vi "Main.vi"() -> ()   [LabVIEW 2020, in "Application.lvlib"]
doc: "This VI is the main application VI in the Delacor QMH project template. This application VI is implemented as a simple state machine, which communicates with two different Delacor QMH modules.\n_____\nBased on DQMH Project Template 6.1.0.93."
uses:
  Application.lvlib
  Application Data--cluster.ctl
  State--enum.ctl
  <vilib>/Utility/error.llb/DialogType.ctl
  Cloneable Module/Cloneable Module.lvlib
  Singleton Module/Singleton Module.lvlib
panel:
  in  "About DQMH":bool
  out "version":string
  in  "Hide Singleton Module Module":bool
  in  "Show Singleton Module Module":bool
  in  "Hide Cloneable Module Module":bool
  in  "Show Cloneable Module Module":bool
  in  "Stop Cloneable Module Module":bool
  in  "Stop Singleton Module Module":bool
  in  "Start Singleton Module Module":bool
  out "Active Cloneable Module Modules":string[](array[string])
  in  "Start New Instance Cloneable Module Module":bool
  in  "Select Cloneable Module Module Instance":i32(ring)=-1 items=["All"=-1, "1"=1]
  in  "Singleton Module Module: Do Something Else":dbl caption="Do Something Else"
  in  "Singleton Module Module: Do Something":bool
  out "Singleton Module Running?":bool
  out "Status":string
  in  "Cloneable Module Module: Do Something Else":dbl caption="Do Something Else to Selected Module"
  in  "Cloneable Module Module: Do Something":bool caption="Do Something to Selected Module"
  # "This top-level application allows you to launch and control a singleton module, and multiple instances of a cloneable module."
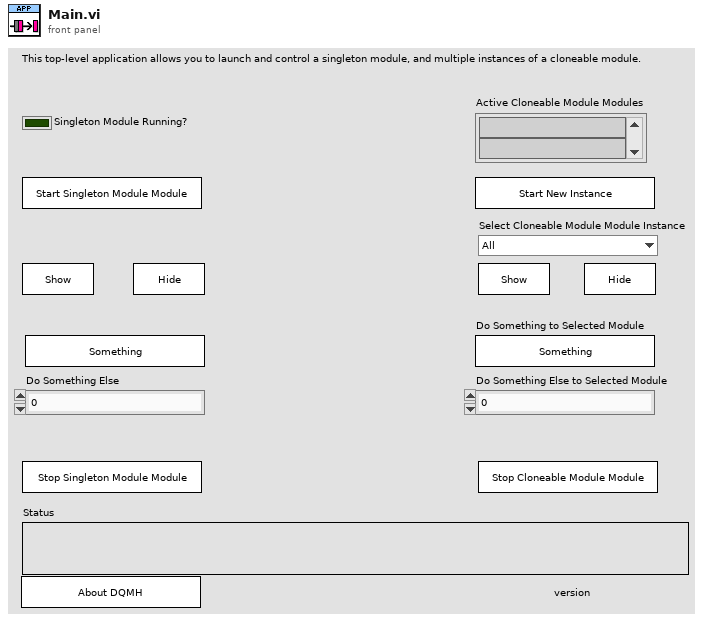
[diagram p1: front panel]
types:
  T1 = typedef "Application.lvlib/State--enum.ctl" = enum16{"Initialize", "Initialize Panel", "UI Interlocks", "Update Status", "Wait for Event", "Exit"}
  T2 = typedef "Application.lvlib/Application Data--cluster.ctl" = cluster{"Status":string, "Singleton Controls":refnum<vi>[], "Cloneable Controls":refnum<vi>[], "Module Ring Value":i32}
  T3 = typedef "Cloneable Module.lvlib/Broadcast Events--cluster.ctl" = cluster{"Module Did Init":refnum<user-event>, "Status Updated":refnum<user-event>, "Error Reported":refnum<user-event>, "Did Something":refnum<user-event>, "Module Did Stop":refnum<user-event>, "Update Module Execution Status":refnum<user-event>}
  T4 = typedef "Singleton Module.lvlib/Broadcast Events--cluster.ctl" = cluster{"Module Did Init":refnum<user-event>, "Status Updated":refnum<user-event>, "Error Reported":refnum<user-event>, "Did Something":refnum<user-event>, "Module Did Stop":refnum<user-event>, "Update Module Execution Status":refnum<user-event>}
  T5 = enum8{"Enabled", "Disabled", "Disabled and Grayed Out"}
  T6 = typedef "DialogType.ctl" = u16
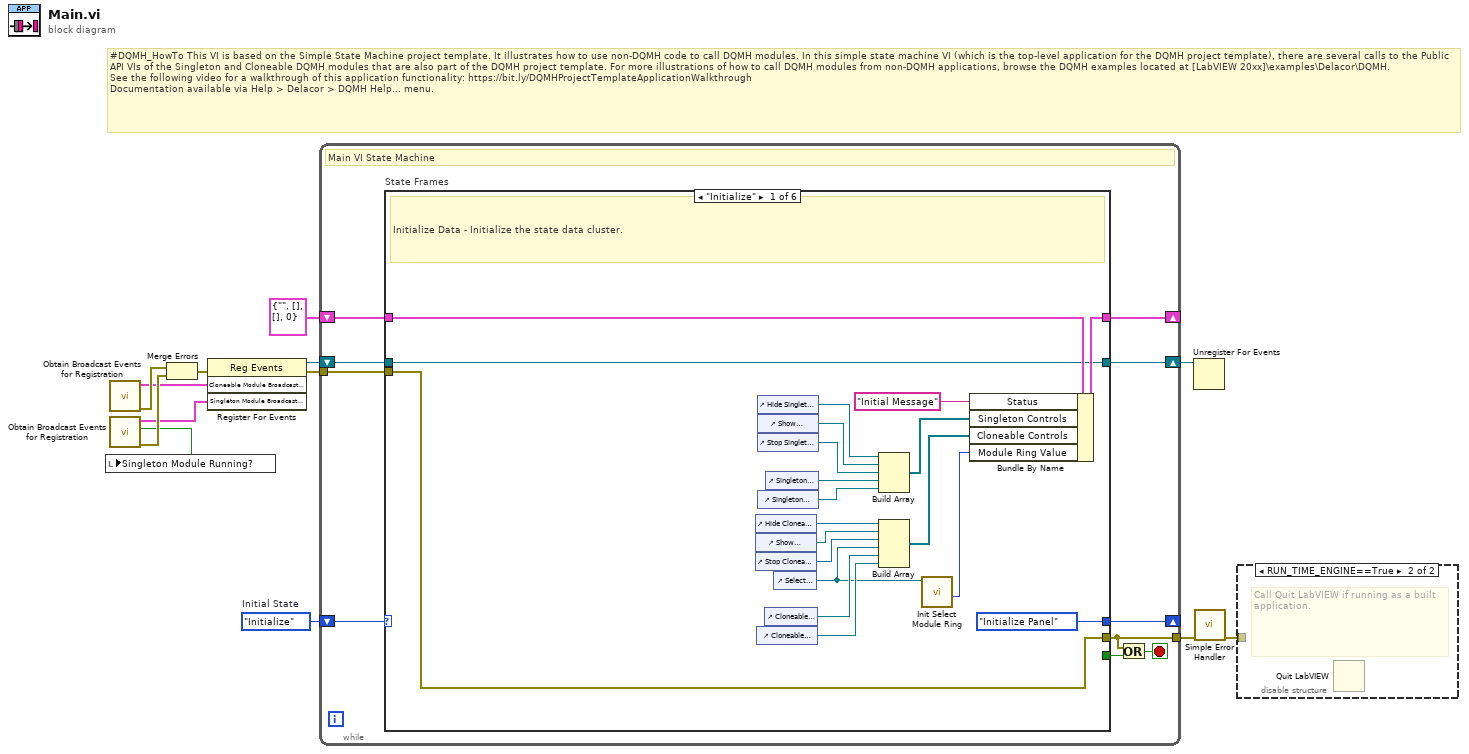
[diagram p0: block diagram]
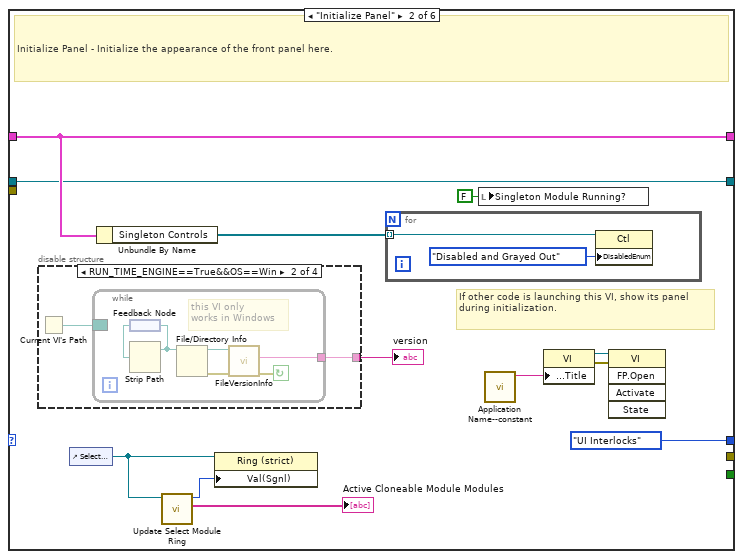
[diagram p2: hidden frame]
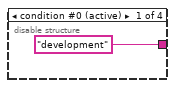
[diagram p3: hidden frame]
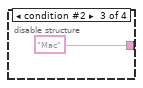
[diagram p4: hidden frame]
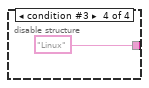
[diagram p5: hidden frame]
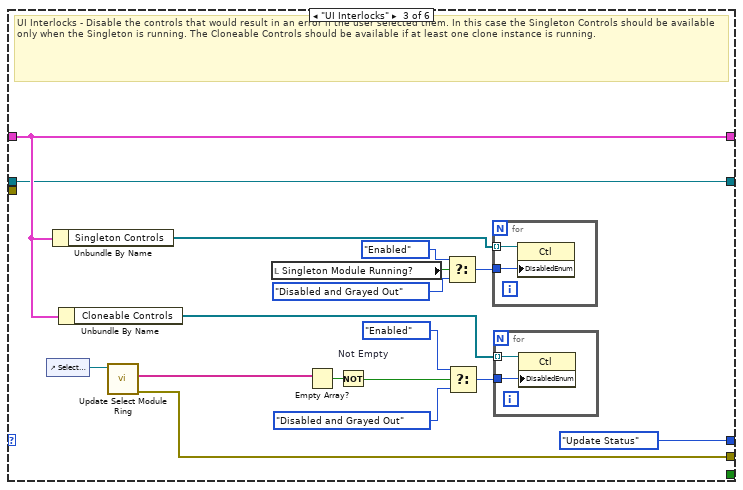
[diagram p6: hidden frame]
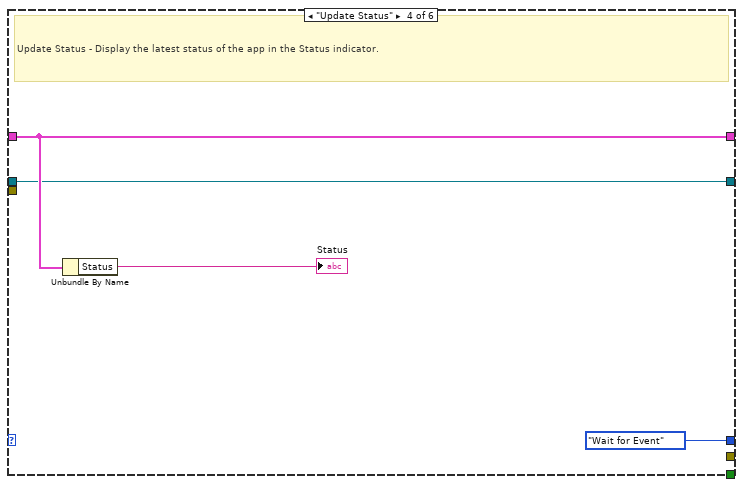
[diagram p7: hidden frame]
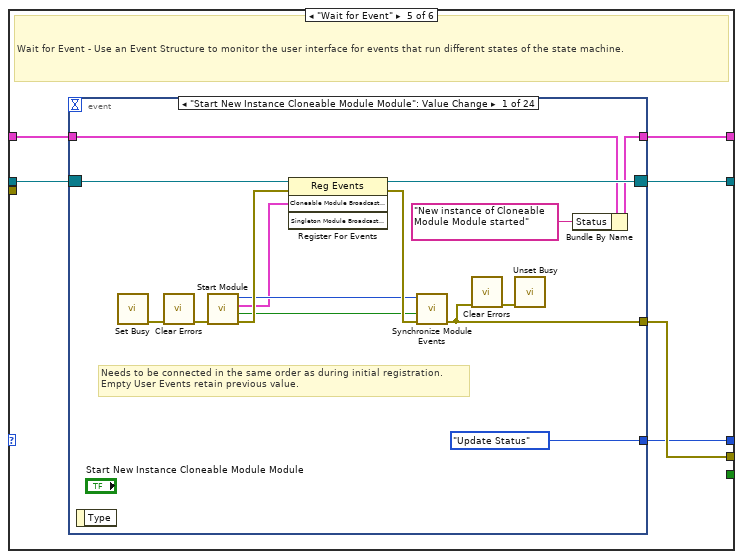
[diagram p8: hidden frame]
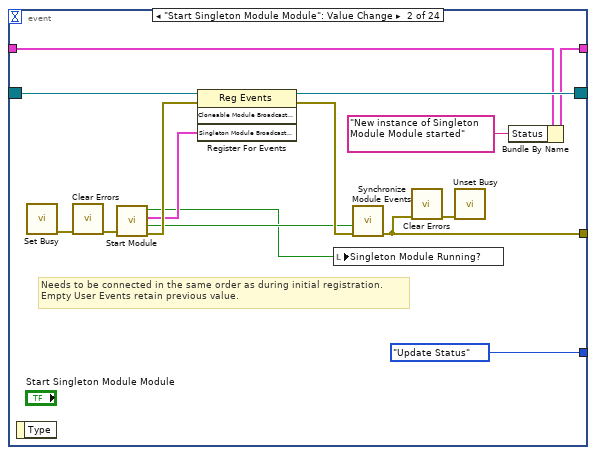
[diagram p9: hidden frame]
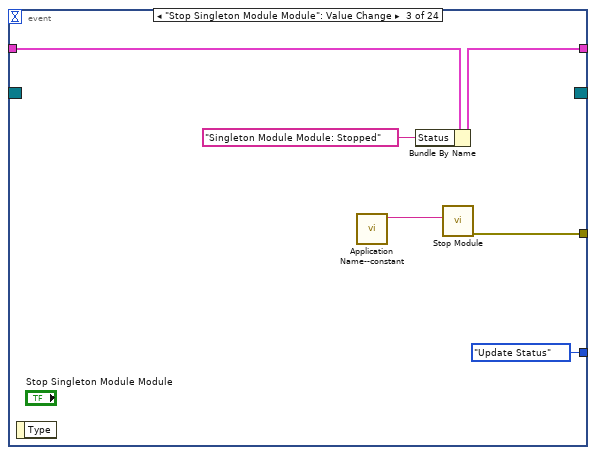
[diagram p10: hidden frame]
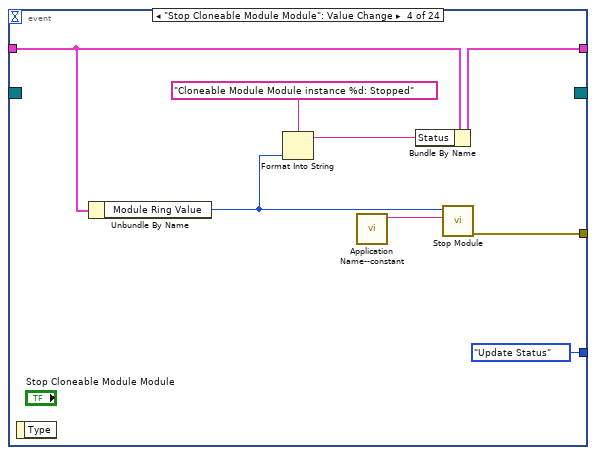
[diagram p11: hidden frame]
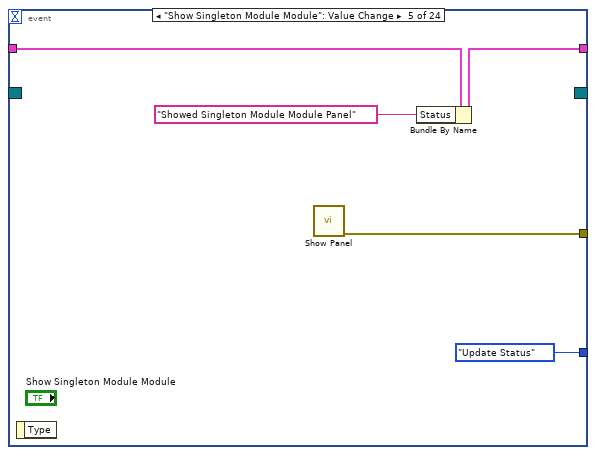
[diagram p12: hidden frame]
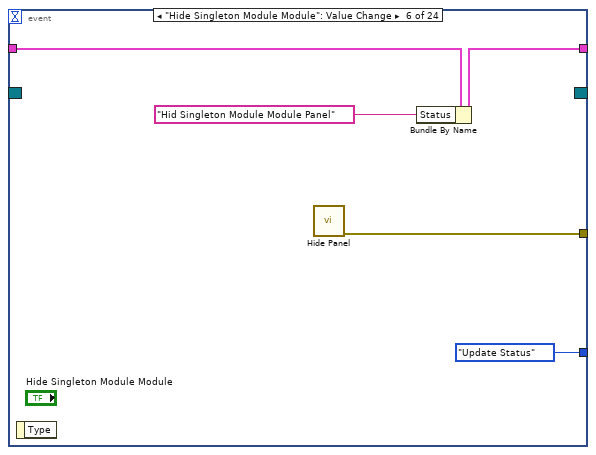
[diagram p13: hidden frame]
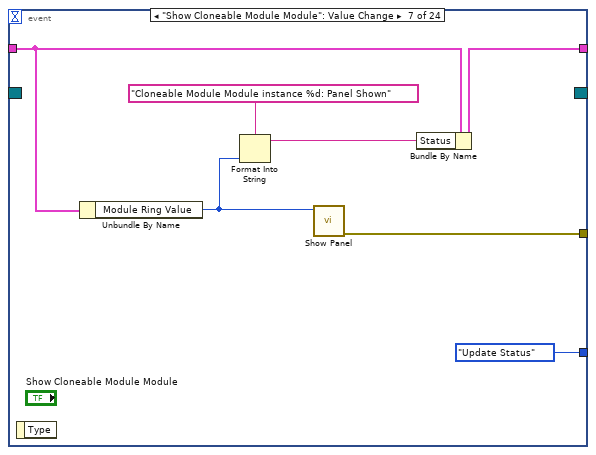
[diagram p14: hidden frame]
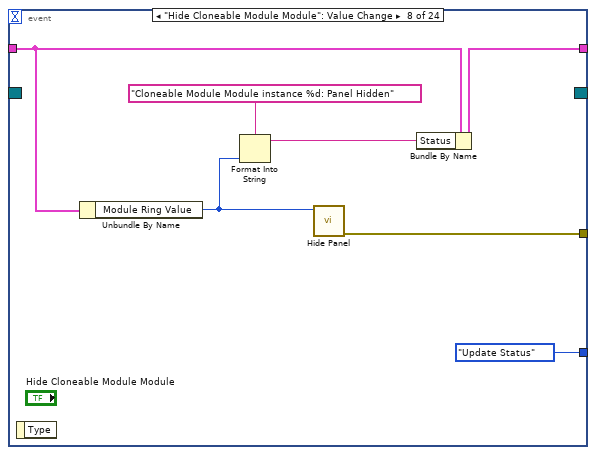
[diagram p15: hidden frame]
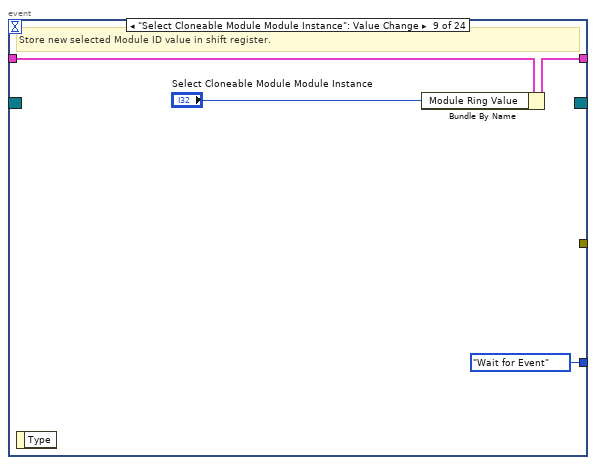
[diagram p16: hidden frame]
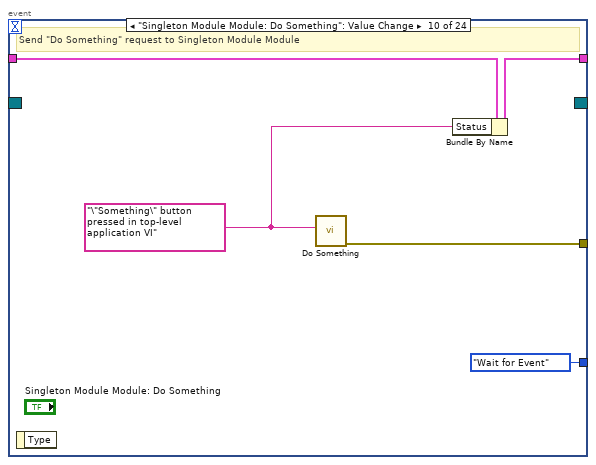
[diagram p17: hidden frame]
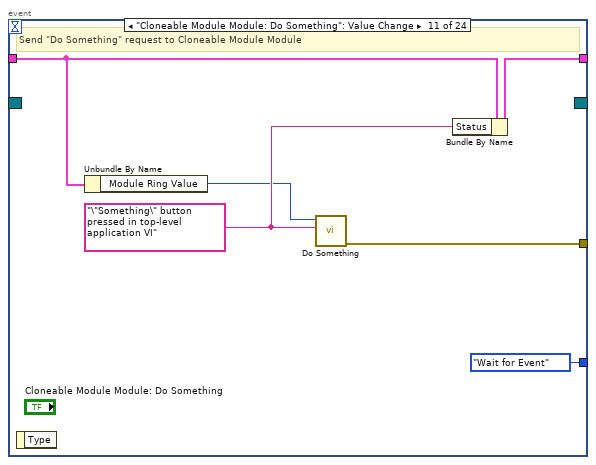
[diagram p18: hidden frame]
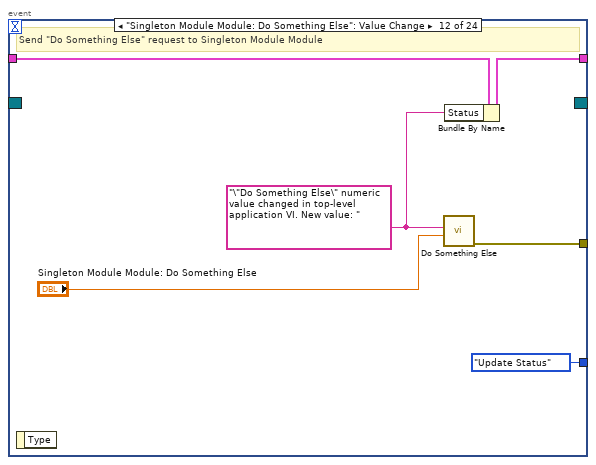
[diagram p19: hidden frame]
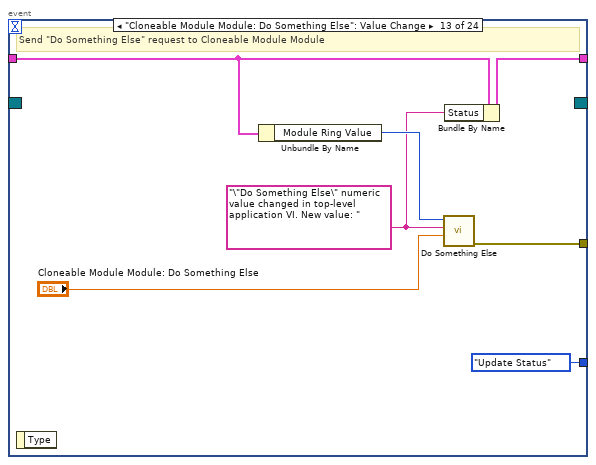
[diagram p20: hidden frame]
diagram:
  w4 = State--enum."Initialize"  # Initial State
  # "#DQMH_HowTo This VI is based on the Simple State Machine project template. It illustrates how to use non-DQMH code to call DQMH modules. In this simple state machine VI (which is the top-level application for the DQMH project template), there are several calls to the Public API VIs of the Singleton and Cloneable DQMH modules that are also part of the DQMH project template. For more illustrations of how to call DQMH modules from non-DQMH applications, browse the DQMH examples located at [LabVIEW 20xx]\\examples\\Delacor\\DQMH.\nSee the following video for a walkthrough of this application functionality: https://bit.ly/DQMHProjectTemplateApplicationWalkthrough\nDocumentation available via Help > Delacor > DQMH Help... menu."
  n1 = call "Obtain Broadcast Events for Registration.vi"() -> ("error out"=w9:errorcluster, "Cloneable Module Broadcast Events"=w6:T3)  [unwired: 9 in, 1 out]
  n2 = call "Obtain Broadcast Events for Registration.vi"() -> ("error out"=w8:errorcluster, "Already running?"=w1:bool, "Singleton Module Broadcast Events"=w5:T4)  [unwired: 9 in]
  n3 = local write "Singleton Module Running?"(w1) -> ()
  n4 = Merge Errors(w9, w8) -> (w10:errorcluster)
  n5 = register-events(error in=w10, w6, w5) -> (reference out=w3:refnum<event-registration>, error out=w11:errorcluster)  [unwired: 1 in]
  n6 = while {
    shift-right: [w20] -> _
    shift-left: T2 {"Status"="", "Singleton Controls"=[], "Cloneable Controls"=[], "Module Ring Value"=0} ("Data Cluster") -> [w21]
    tunnel: [w23] -> w13
    shift-right: [w16] -> _
    shift-left: w4 -> [w18]
    shift-right: [w14] -> w2
    shift-left: w3 -> [w15]
    tunnel: w11 -> [w22]
    stop <- w17 stop-if-true
    # "Main VI State Machine"
    n7 = case "State Frames" shown="\"Initialize\"" w18 {
      tunnel: [w43 _ w85 _ w99 w277] -> w23
      tunnel: w21 -> [w42 w52 w73 w93 w96 w274]
      tunnel: [w41 w52 w73 w93 w95 w274] -> w20
      tunnel: [_ _ _ _ _ w273] -> w19
      tunnel: [State--enum."Initialize Panel" ("State") State--enum."UI Interlocks" ("State") State--enum."Update Status" ("State") State--enum."Wait for Event" ("State") w94 State--enum."Exit" ("State")] -> w16
      tunnel: w15 -> [w24 w49 w69 w90 w98 w271]
      tunnel: [w24 w49 w69 w90 w97 w271] -> w14
      tunnel: w22 -> [w43 _ _ _ _ _]
      frame "Initialize" {
        # "Initialize Data - Initialize the state data cluster."
        n8 = control-ref of="Hide Cloneable Module Module"() -> (w33:refnum<vi>)
        n9 = control-ref of="Show Cloneable Module Module"() -> (w32:refnum<vi>)
        n10 = control-ref of="Stop Cloneable Module Module"() -> (w31:refnum<vi>)
        n11 = control-ref of="Cloneable Module Module: Do Something"() -> (w28:refnum<vi>)
        n12 = control-ref of="Hide Singleton Module Module"() -> (w39:refnum<vi>)
        n13 = control-ref of="Show Singleton Module Module"() -> (w38:refnum<vi>)
        n14 = control-ref of="Stop Singleton Module Module"() -> (w37:refnum<vi>)
        n15 = control-ref of="Singleton Module Module: Do Something"() -> (w35:refnum<vi>)
        n16 = control-ref of="Cloneable Module Module: Do Something Else"() -> (w29:refnum<vi>)
        n17 = control-ref of="Singleton Module Module: Do Something Else"() -> (w36:refnum<vi>)
        n18 = control-ref of="Select Cloneable Module Module Instance"() -> (w26:refnum<vi>)
        n19 = Build Array(w39, w38, w37, w36, w35) -> (w34:refnum<vi>[])
        n20 = Build Array(w33, w32, w31, w26, w29, w28) -> (w30:refnum<vi>[])
        n21 = call "Init Select Module Ring.vi"("Select Module Ring Ref"=w26) -> ("Module Ring Value"=w25:i32)  [unwired: 8 in, 2 out]
        n22 = Bundle By Name(cluster=w42, "Status"="Initial Message" ("Initial Message"), "Singleton Controls"=w34, "Cloneable Controls"=w30, "Module Ring Value"=w25) -> (w41:T2)
      }
      frame "Initialize Panel" {
        # "If other code is launching this VI, show its panel during initialization."
        # "Initialize Panel - Initialize the appearance of the front panel here."
        n23 = disable-structure "Conditional Disable Structure" shown="RUN_TIME_ENGINE==True&&OS==Win" {
          disable-tunnel: ["development" w57 "Mac" "Linux"] -> w46
          frame condition #0 (active) {
          }
          frame condition #1 {
            n24 = Current VI's Path() -> (path=w58:path)
            n25 = while {
              border: w58 -> [_]
              tunnel: [w59] -> w57
              stop <- w63 continue-if-true
              # "this VI only \nworks in Windows"
              n26 = feedback #1() -> (w62:path)
              n27 = Strip Path(path=w62) -> (stripped path=w61:path)  [unwired: 1 out]
              n28 = feedback-in #1(w61) -> ()
              n29 = File/Directory Info(path=w61) -> (path out=w60:path, error out=w64:errorcluster)  [unwired: 1 in, 5 out]
              n30 = call <vilib>:"FileVersionInfo.vi"("error in (no error)"=w64, "Application Path in"=w60) -> ("error out"=w63:errorcluster, "File Version Info"=w59:string)  [unwired: 6 in, 2 out]
            }
          }
          frame condition #2 {
          }
          frame condition #3 {
          }
        }
        "version" <- w46
        n31 = control-ref of="Select Cloneable Module Module Instance"() -> (w48:refnum<vi>)
        n32 = Unbundle By Name(w52) -> ("Singleton Controls"=w51:refnum<vi>[])
        n33 = call "Update Select Module Ring.vi"("Select Module Ring Ref"=w48) -> ("Active Modules (Array)"=→"Active Cloneable Module Modules":string[], "New Module Ring Value"=w47:i32)  [unwired: 8 in, 1 out]
        n34 = property on="Property Node" class="Ring (strict)"(reference=w48, "Val(Sgnl)"=w47) -> ()  [unwired: 1 in, 2 out]
        n35 = for {
          tunnel: w51 -> [w68] mode=indexing
          n36 = property on="Property Node" class="Ctl"(reference=w68, "DisabledEnum"=T5."Disabled and Grayed Out" ("Disabled")) -> ()  [unwired: 1 in, 2 out]
        }
        n37 = local write "Singleton Module Running?"(FALSE ("My Singleton Module Init?")) -> ()
        n38 = call "Application Name--constant.vi"() -> ("Application Name"=w45:string)  [unwired: 11 in]
        n39 = property on="Property Node" class="VI"("Front Panel.Title"=w45) -> (reference out=w44:refnum<vi>, error out=w55:errorcluster)  [unwired: 2 in]
        n40 = invoke class="VI" method="FP.Open"(reference=w44, error in=w55) -> ()  [unwired: 3 in, 5 out]
      }
      frame "UI Interlocks" {
        # "UI Interlocks - Disable the controls that would result in an error if the user selected them. In this case the Singleton Controls should be available only when the Singleton is running. The Cloneable Controls should be available if at least one clone instance is running."
        n41 = control-ref of="Select Cloneable Module Module Instance"() -> (w84:refnum<vi>)
        n42 = Unbundle By Name(w73) -> ("Singleton Controls"=w78:refnum<vi>[])
        n43 = Unbundle By Name(w73) -> ("Cloneable Controls"=w72:refnum<vi>[])
        n44 = call "Update Select Module Ring.vi"("Select Module Ring Ref"=w84) -> ("error out"=w85:errorcluster, "Active Modules (Array)"=w83:string[])  [unwired: 8 in, 1 out]
        n45 = local read "Singleton Module Running?"() -> (w77:bool)
        n46 = Empty Array?(array=w83) -> (empty?=w82:bool)
        n47 = Not "Not Empty"(x=w82) -> (.not. x?=w71:bool)
        n48 = Select(t=T5."Enabled" ("Disabled"), s=w77, f=T5."Disabled and Grayed Out" ("Disabled")) -> (s? t:f=w79:T5)
        n49 = Select(t=T5."Enabled" ("Disabled"), s=w71, f=T5."Disabled and Grayed Out" ("Disabled")) -> (s? t:f=w76:T5)
        n50 = for {
          tunnel: w78 -> [w89] mode=indexing
          tunnel: w79 -> [w88]
          n51 = property on="Property Node" class="Ctl"(reference=w89, "DisabledEnum"=w88) -> ()  [unwired: 1 in, 2 out]
        }
        n52 = for {
          tunnel: w72 -> [w87] mode=indexing
          tunnel: w76 -> [w86]
          n53 = property on="Property Node" class="Ctl"(reference=w87, "DisabledEnum"=w86) -> ()  [unwired: 1 in, 2 out]
        }
      }
      frame "Update Status" {
        # "Update Status - Display the latest status of the app in the Status indicator."
        n54 = Unbundle By Name(w93) -> ("Status"=→"Status":string)
      }
      frame "Wait for Event" {
        # "Wait for Event - Use an Event Structure to monitor the user interface for events that run different states of the state machine."
        n55 = event shown="[0] \"Start New Instance Cloneable Module Module\": Value Change" {
          selector: w98 -> [w106 w122 _ _ _ _ _ _ _ _ _ _ _ _ _ _ _ _ _ _ _ _ _ _]
          dyn-events: [w105 w121 _ _ _ _ _ _ _ _ _ _ _ _ _ _ _ _ _ _ _ _ _ _] -> w97
          timeout: _ -> [_ _ _ _ _ _ _ _ _ _ _ _ _ _ _ _ _ _ _ _ _ _ _ _]
          tunnel: [w114 w129 w135 w143 w148 w153 w160 w167 _ w176 w182 w188 w195 w203 w208 w212 _ _ _ _ w254 _ _ w265] -> w99
          tunnel: [w101 w118 w131 w140 w146 w151 w159 w166 w169 w174 w181 w186 w194 w197 w205 w211 w214 w219 w234 w243 w247 w258 w263 w267] -> w95
          tunnel: w96 -> [w102 w119 w132 w139 w147 w152 w157 w164 w170 w175 w178 w187 w192 w197 w205 w211 w215 w220 w235 w244 w250 w259 w263 w267]
          tunnel: [State--enum."Update Status" ("State") State--enum."Update Status" ("State") State--enum."Update Status" ("State") State--enum."Update Status" ("State") State--enum."Update Status" ("State") State--enum."Update Status" ("State") State--enum."Update Status" ("State") State--enum."Update Status" ("State") State--enum."Wait for Event" ("State") State--enum."Wait for Event" ("State") State--enum."Wait for Event" ("State") State--enum."Update Status" ("State") State--enum."Update Status" ("State") State--enum."UI Interlocks" ("State") State--enum."UI Interlocks" ("State") State--enum."UI Interlocks" ("State") State--enum."Update Status" ("State") State--enum."Update Status" ("State") State--enum."Update Status" ("State") State--enum."Update Status" ("State") State--enum."UI Interlocks" ("State") State--enum."UI Interlocks" ("State") State--enum."Exit" ("State") State--enum."Wait for Event" ("State")] -> w94
          event "Start New Instance Cloneable Module Module": Value Change {
            # "Needs to be connected in the same order as during initial registration.\nEmpty User Events retain previous value."
            n56 = event-data() -> ()  [unwired: 1 in, 1 out]
            n57 = call <vilib>:"Set Busy.vi"() -> ("error out"=w110:errorcluster)  [unwired: 10 in, 1 out]
            n58 = call <vilib>:"Clear Errors.vi"("error in (no error)"=w110) -> ("error out"=w111:errorcluster)  [unwired: 5 in, 1 out]
            n59 = call "Start Module.vi"("error in"=w111) -> ("error out"=w113:errorcluster, "Wait for Event Sync?"=w108:bool, "Cloneable Module Broadcast Events"=w104:T3, "Module ID"=w107:i32)  [unwired: 7 in]
            n60 = register-events(reference=w106, error in=w113, w104) -> (reference out=w105:refnum<event-registration>, error out=w112:errorcluster)  [unwired: 1 in]
            n61 = call "Synchronize Module Events.vi"("error in"=w112, "Wait for Event Sync?"=w108, "Module ID in"=w107) -> ("error out"=w114:errorcluster)  [unwired: 7 in, 1 out]
            n62 = call <vilib>:"Clear Errors.vi"("error in (no error)"=w114) -> ("error out"=w109:errorcluster)  [unwired: 5 in, 1 out]
            n63 = call <vilib>:"Unset Busy.vi"("error in (no error)"=w109) -> ()  [unwired: 10 in, 1 out]
            n64 = Bundle By Name(cluster=w102, "Status"="New instance of Cloneable Module Module started") -> (w101:T2)
          }
          event "Start Singleton Module Module": Value Change {
            # "Needs to be connected in the same order as during initial registration.\nEmpty User Events retain previous value."
            n65 = event-data() -> ()  [unwired: 1 in, 1 out]
            n66 = call <vilib>:"Set Busy.vi"() -> ("error out"=w125:errorcluster)  [unwired: 10 in, 1 out]
            n67 = call <vilib>:"Clear Errors.vi"("error in (no error)"=w125) -> ("error out"=w126:errorcluster)  [unwired: 5 in, 1 out]
            n68 = call "Start Module.vi"("error in"=w126) -> ("error out"=w128:errorcluster, "Wait for Event Sync?"=w123:bool, "Singleton Module Broadcast Events"=w116:T4, "Module Was Already Running?"=w115:bool)  [unwired: 7 in]
            n69 = register-events(reference=w122, error in=w128, w116) -> (reference out=w121:refnum<event-registration>, error out=w127:errorcluster)  [unwired: 1 in]
            n70 = local write "Singleton Module Running?"(w115) -> ()
            n71 = call "Synchronize Module Events.vi"("error in"=w127, "Wait for Event Sync?"=w123) -> ("error out"=w129:errorcluster)  [unwired: 9 in]
            n72 = call <vilib>:"Clear Errors.vi"("error in (no error)"=w129) -> ("error out"=w124:errorcluster)  [unwired: 5 in, 1 out]
            n73 = call <vilib>:"Unset Busy.vi"("error in (no error)"=w124) -> ()  [unwired: 10 in, 1 out]
            n74 = Bundle By Name(cluster=w119, "Status"="New instance of Singleton Module Module started") -> (w118:T2)
          }
          event "Stop Singleton Module Module": Value Change {
            n75 = event-data() -> ()  [unwired: 1 in, 1 out]
            n76 = call "Application Name--constant.vi"() -> ("Application Name"=w133:string)  [unwired: 11 in]
            n77 = Bundle By Name(cluster=w132, "Status"="Singleton Module Module: Stopped" ("Message")) -> (w131:T2)
            n78 = call "Stop Module.vi"("Origin"=w133) -> ("error out"=w135:errorcluster)  [unwired: 10 in]
          }
          event "Stop Cloneable Module Module": Value Change {
            n79 = event-data() -> ()  [unwired: 1 in, 1 out]
            n80 = Unbundle By Name(w139) -> ("Module Ring Value"=w136:i32)
            n81 = Format Into String(format string="Cloneable Module Module instance %d: Stopped" ("Message"), w136) -> (resulting string=w137:string)  [unwired: 2 in, 1 out]
            n82 = call "Application Name--constant.vi"() -> ("Application Name"=w141:string)  [unwired: 11 in]
            n83 = Bundle By Name(cluster=w139, "Status"=w137) -> (w140:T2)
            n84 = call "Stop Module.vi"("Origin"=w141, "Module ID"=w136) -> ("error out"=w143:errorcluster)  [unwired: 9 in]
          }
          event "Show Singleton Module Module": Value Change {
            n85 = event-data() -> ()  [unwired: 1 in, 1 out]
            n86 = call "Show Panel.vi"() -> ("error out"=w148:errorcluster)  [unwired: 11 in]
            n87 = Bundle By Name(cluster=w147, "Status"="Showed Singleton Module Module Panel" ("Message")) -> (w146:T2)
          }
          event "Hide Singleton Module Module": Value Change {
            n88 = event-data() -> ()  [unwired: 1 in, 1 out]
            n89 = call "Hide Panel.vi"() -> ("error out"=w153:errorcluster)  [unwired: 11 in]
            n90 = Bundle By Name(cluster=w152, "Status"="Hid Singleton Module Module Panel" ("Message")) -> (w151:T2)
          }
          event "Show Cloneable Module Module": Value Change {
            n91 = event-data() -> ()  [unwired: 1 in, 1 out]
            n92 = Unbundle By Name(w157) -> ("Module Ring Value"=w155:i32)
            n93 = Format Into String(format string="Cloneable Module Module instance %d: Panel Shown" ("Message"), w155) -> (resulting string=w154:string)  [unwired: 2 in, 1 out]
            n94 = call "Show Panel.vi"("Module ID"=w155) -> ("error out"=w160:errorcluster)  [unwired: 10 in]
            n95 = Bundle By Name(cluster=w157, "Status"=w154) -> (w159:T2)
          }
          event "Hide Cloneable Module Module": Value Change {
            n96 = event-data() -> ()  [unwired: 1 in, 1 out]
            n97 = Unbundle By Name(w164) -> ("Module Ring Value"=w162:i32)
            n98 = Format Into String(format string="Cloneable Module Module instance %d: Panel Hidden" ("Message"), w162) -> (resulting string=w161:string)  [unwired: 2 in, 1 out]
            n99 = call "Hide Panel.vi"("Module ID"=w162) -> ("error out"=w167:errorcluster)  [unwired: 10 in]
            n100 = Bundle By Name(cluster=w164, "Status"=w161) -> (w166:T2)
          }
          event "Select Cloneable Module Module Instance": Value Change {
            # "Store new selected Module ID value in shift register."
            n101 = event-data() -> ()  [unwired: 1 in, 1 out]
            n102 = Bundle By Name(cluster=w170, "Module Ring Value"="Select Cloneable Module Module Instance") -> (w169:T2)
          }
          event "Singleton Module Module: Do Something": Value Change {
            w173 = "\"Something\" button pressed in top-level application VI" ("\"Do Something Else\" button pressed")
            # "Send \"Do Something\" request to Singleton Module Module"
            n103 = event-data() -> ()  [unwired: 1 in, 1 out]
            n104 = call "Do Something.vi"("Do Something Message"=w173) -> ("error out"=w176:errorcluster)  [unwired: 10 in]
            n105 = Bundle By Name(cluster=w175, "Status"=w173) -> (w174:T2)
          }
          event "Cloneable Module Module: Do Something": Value Change {
            w180 = "\"Something\" button pressed in top-level application VI" ("\"Do Something Else\" button pressed")
            # "Send \"Do Something\" request to Cloneable Module Module"
            n106 = event-data() -> ()  [unwired: 1 in, 1 out]
            n107 = Unbundle By Name(w178) -> ("Module Ring Value"=w177:i32)
            n108 = call "Do Something.vi"("Do Something Message"=w180, "Module ID"=w177) -> ("error out"=w182:errorcluster)  [unwired: 9 in]
            n109 = Bundle By Name(cluster=w178, "Status"=w180) -> (w181:T2)
          }
          event "Singleton Module Module: Do Something Else": Value Change {
            w183 = "\"Do Something Else\" numeric value changed in top-level application VI. New value: " ("\"Do Something Else\" button pressed")
            # "Send \"Do Something Else\" request to Singleton Module Module"
            n110 = event-data() -> ()  [unwired: 1 in, 1 out]
            n111 = call "Do Something Else.vi"("X"="Singleton Module Module: Do Something Else", "Do Something Else Message"=w183) -> ("error out"=w188:errorcluster)  [unwired: 9 in]
            n112 = Bundle By Name(cluster=w187, "Status"=w183) -> (w186:T2)
          }
          event "Cloneable Module Module: Do Something Else": Value Change {
            w189 = "\"Do Something Else\" numeric value changed in top-level application VI. New value: " ("\"Do Something Else\" button pressed")
            # "Send \"Do Something Else\" request to Cloneable Module Module"
            n113 = event-data() -> ()  [unwired: 1 in, 1 out]
            n114 = Unbundle By Name(w192) -> ("Module Ring Value"=w191:i32)
            n115 = call "Do Something Else.vi"("X"="Cloneable Module Module: Do Something Else", "Do Something else Message"=w189, "Module ID"=w191) -> ("error out"=w195:errorcluster)  [unwired: 8 in]
            n116 = Bundle By Name(cluster=w192, "Status"=w189) -> (w194:T2)
          }
          event User Event {
            # "A new instance of Cloneable Module Module has broadcast that is has been initialized"
            n117 = event-data() -> ("Info"=w201:string, "Module ID"=w196:i32)  [unwired: 1 in]
            n118 = local write "Status"(w201) -> ()
            n119 = control-ref of="Select Cloneable Module Module Instance"() -> (w200:refnum<vi>)
            n120 = call "Update Select Module Ring.vi"("Select Module Ring Ref"=w200) -> ("error out"=w202:errorcluster, "Active Modules (Array)"=w199:string[])  [unwired: 8 in, 1 out]
            n121 = local write "Active Cloneable Module Modules"(w199) -> ()
            n122 = call "Show Panel.vi"("error in (no error)"=w202, "Module ID"=w196) -> ("error out"=w203:errorcluster)  [unwired: 9 in]
          }
          event User Event {
            # "Singleton Module Module has broadcast that it has been initialized"
            n123 = event-data() -> ("Init?"=→"Singleton Module Running?":bool, "Info"=w207:string)  [unwired: 1 in]
            n124 = local write "Status"(w207) -> ()
            n125 = call "Show Panel.vi"() -> ("error out"=w208:errorcluster)  [unwired: 11 in]
          }
          event User Event {
            # "Singleton Module Module has broadcast its execution status"
            n126 = event-data() -> ("Running?"=w209:bool)  [unwired: 1 in]
            n127 = local write "Singleton Module Running?"(w209) -> ()
            n128 = case shown="True" w209 {
              tunnel: [_ w213] -> w212
              frame False {
              }
              frame True {
                n129 = call "Show Panel.vi"() -> ("error out"=w213:errorcluster)  [unwired: 11 in]
              }
            }
          }
          event User Event {
            # "An instance of Cloneable Module Module has broadcast its status"
            n130 = event-data() -> ("Status"=w217:string)  [unwired: 1 in]
            n131 = Bundle By Name(cluster=w215, "Status"=w217) -> (w214:T2)
          }
          event User Event {
            # "Singleton Module Module has broadcast its status"
            n132 = event-data() -> ("Status"=w221:string)  [unwired: 1 in]
            n133 = Bundle By Name(cluster=w220, "Status"=w221) -> (w219:T2)
          }
          event User Event {
            w226 = T6 0 items=["no dialog", "OK message", "continue or stop message", "OK message + warnings", "continue/stop + warnings"] ("type of dialog (OK msg:1)")
            # "Cloneable Module Module had an error"
            n134 = event-data() -> ("Module Name"=w223:string, "Additional Information"=w224:string, "Error"=w225:errorcluster)  [unwired: 1 in]
            n135 = call <vilib>:"Space Constant.vi"() -> ("String"=w230:string)
            n136 = call <vilib>:"Simple Error Handler.vi"("type of dialog (OK msg:1)"=w226, "error in (no error)"=w225) -> ("message"=w227:string)  [unwired: 3 in, 4 out]
            n137 = call <vilib>:"Search and Replace Pattern.vi"("string"=w227, "regular expression (\"\")"="[\\r\\n]" ("regular expression (\"\")"), "replace string (\"\")"=w230, "replace all? (F)"=TRUE ("replace all CR/LF with spaces")) -> ("result string"=w228:string)  [unwired: 1 in, 1 out]
            n138 = Format Into String(format string="%s: %s Additional Information: %s", w223, w228, w224) -> (resulting string=w222:string)  [unwired: 2 in, 1 out]
            n139 = Bundle By Name(cluster=w235, "Status"=w222) -> (w234:T2)
          }
          event User Event {
            # "Singleton Module Module had an error"
            n140 = event-data() -> ("Module Name"=w237:string, "Additional Information"=w241:string, "Error"=w245:errorcluster)  [unwired: 1 in]
            n141 = Unbundle By Name(w245) -> ("code"=w236:i32, "source"=w240:string)
            n142 = Format Into String(format string="Error code %d Module: %s  Additional Information: %s\nSource: %s", w236, w237, w241, w240) -> (resulting string=w238:string)  [unwired: 2 in, 1 out]
            n143 = Bundle By Name(cluster=w244, "Status"=w238) -> (w243:T2)
          }
          event User Event {
            n144 = event-data() -> ("Origin"=w249:string)  [unwired: 1 in]
            n145 = Bundle By Name(cluster=w250, "Status"=w249) -> (w248:T2)
            n146 = control-ref of="Select Cloneable Module Module Instance"() -> (w253:refnum<vi>)
            n147 = call "Update Select Module Ring.vi"("Select Module Ring Ref"=w253) -> ("error out"=w254:errorcluster, "Active Modules (Array)"=w252:string[], "New Module Ring Value"=w246:i32)  [unwired: 8 in]
            n148 = local write "Active Cloneable Module Modules"(w252) -> ()
            n149 = Bundle By Name(cluster=w248, "Module Ring Value"=w246) -> (w247:T2)
          }
          event User Event {
            n150 = event-data() -> ("Origin"=w256:string)  [unwired: 1 in]
            n151 = local write "Singleton Module Running?"(FALSE ("My Singleton Module Init?")) -> ()
            n152 = Concatenate Strings(w256, " Did Stop.") -> (w255:string)
            n153 = Bundle By Name(cluster=w259, "Status"=w255) -> (w258:T2)
          }
          event Panel Close? {
            # "Go to the 'Exit' state if the user tries to close the panel."
            n154 = event-data() -> ()  [unwired: 1 in, 1 out]
            n155 = event-data ("Event Filter Node")("Discard?"=TRUE) -> ()  [unwired: 1 in, 1 out]
          }
          event "About DQMH": Value Change {
            # "Display DQMH About Box"
            n156 = event-data() -> ()  [unwired: 1 in, 1 out]
            n157 = call <vilib>:"DQMH_About Box.vi"() -> ("error out"=w265:errorcluster)  [unwired: 11 in]
          }
        }
      }
      frame "Exit" {
        w268 = TRUE  # Wait for Module to stop?
        w273 = TRUE  # Stop the VI
        # "Stop all modules launched"
        # "Exit - Exit the application."
        n158 = call "Application Name--constant.vi"() -> ("Application Name"=w269:string)  [unwired: 11 in]
        n159 = call "Stop Module.vi"("Wait for Module to stop? (F)"=w268, "Origin"=w269, "Module ID"=-1) -> ("error out"=w275:errorcluster)  [unwired: 8 in]
        n160 = call "Stop Module.vi"("Wait for Module to Stop? (F)"=w268, "Origin"=w269) -> ("error out"=w276:errorcluster)  [unwired: 9 in]
        n161 = Merge Errors(w275, w276) -> (w277:errorcluster)
      }
    }
    n162 = Or(x=w23, y=w19) -> (x .or. y?=w17:bool)
  }
  n163 = Unregister For Events(event registration refnum=w2) -> ()  [unwired: 1 in, 1 out]
  n164 = call <vilib>:"Simple Error Handler.vi"("error in (no error)"=w13) -> ("error out"=w12:errorcluster)  [unwired: 4 in, 4 out]
  n165 = disable-structure "Conditional Disable Structure" shown="RUN_TIME_ENGINE==True" {
    disable-tunnel: w12 -> [_ _]
    frame condition #0 (active) {
    }
    frame condition #1 {
      # "Call Quit LabVIEW if running as a built application."
      n166 = Quit LabVIEW() -> ()  [unwired: 1 in]
    }
  }
